vi "WriteMotorInformation.vi"(8 "error in (no error)":errorcluster, 10 "Properties":T1[](array[typedef]), 11 "map in":T2) -> (0 "error out":errorcluster, 3 "map out":T2)   [LabVIEW 2017, in "McsaUtilities.lvlib"]
uses:
  <vilib>/addons/InsightCM/Utilities/MCSA/McsaUtilities.lvlib
  <vilib>/addons/PointValueMap/controls/PointMap.ctl
  <vilib>/addons/InsightCM/MessageBus/Base/controls/KeyValuePair.ctl
  <vilib>/addons/PointValueMap/subVIs/Point_Write_variant.vi
  <vilib>/addons/PointValueMap/PointValueMap.lvlib
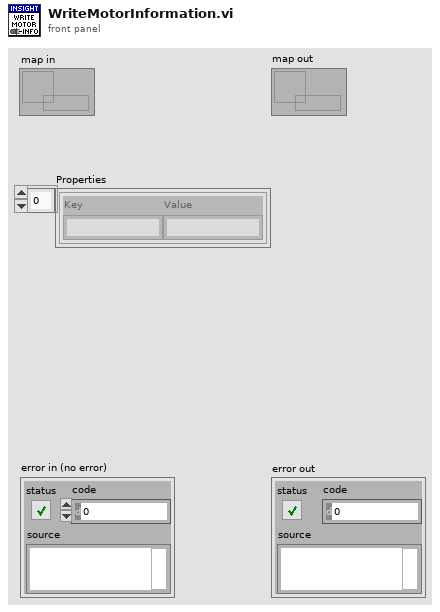
[diagram p1: front panel]
types:
  T1 = typedef "KeyValuePair.ctl" = cluster{"Key":string, "Value":string}
  T2 = typedef "PointValueMap.lvlib/PointMap.ctl" = refnum<data-value>
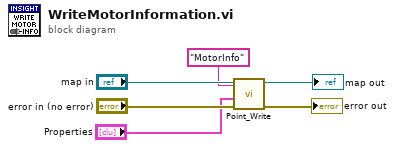
[diagram p0: block diagram]
diagram:
  n1 = call-poly <vilib>:"Point_Write.vi"("Error In"="error in (no error)", "Value"="Properties", "Tag"="MotorInfo", "Map"="map in") -> ("Error Out"=→"error out":errorcluster, "Map Out"=→"map out":T2)  [unwired: 6 in]
